vi "ProcessListGlb.vi"() -> ()   [LabVIEW 2019]
panel:
  out "ProceListPath":path
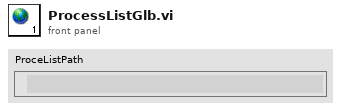
[diagram p1: front panel]
diagram:
